vi "crosscorr_sub2.vi"(0 "reference":refnum<vi>, 1 "B":dbl=500.0 format="%.2f", 5 "binning":refnum<vi>, 7 "macro times 1":i32[](array[numeric]), 9 "macro times 2":i32[](array[numeric]), 11 "cross ch2 (MCS)":i32, 12 "cross ch1 (MCS)":i32, 13 "skip":i32, 14 "biExp fit":bool) -> (6 "crosscorrelation":cluster{"Tau Values":dbl[], "best fit":dbl[]}[](array[cluster]), 8 "F2":dbl, 10 "S+B":dbl, 15 "fit results":cluster{dbl, dbl, dbl, dbl, dbl, dbl})   [LabVIEW 2009]
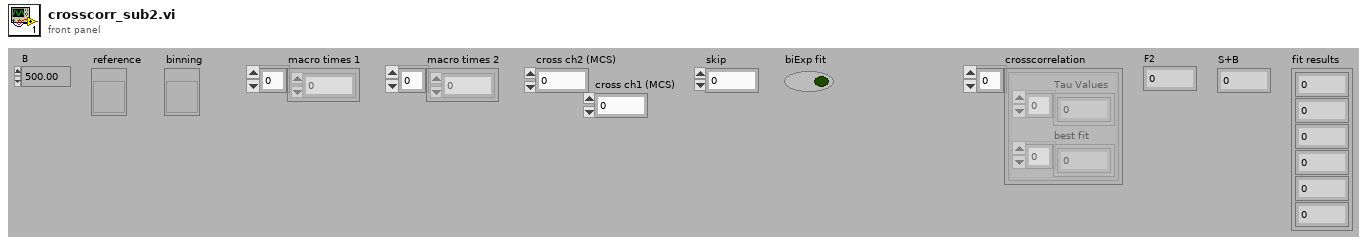
[diagram p1: front panel]
types:
  T1 = cluster{"binning (s)":dbl, "binning (s)":dbl, "Histogram: h(x)":u32[]}[]
  T2 = cluster{"binning (s)":dbl, "binning (s)":dbl, "Histogram: h(x)":u32[]}
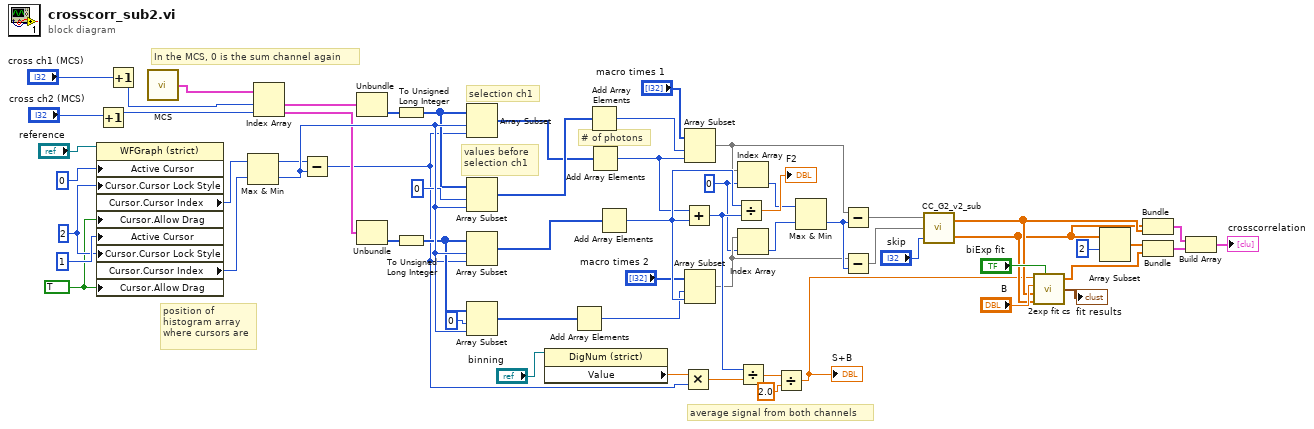
[diagram p0: block diagram]
diagram:
  w39 = 0 ("Index")
  w23 = u32 2 ("Write Attribute")
  w16 = TRUE ("Write Attribute")
  # "average signal from both channels"
  # "In the MCS, 0 is the sum channel again"
  # "# of photons"
  # "values before \nselection ch1"
  # "position of\nhistogram array\nwhere cursors are"
  # "selection ch1"
  n1 = property on="Property Node" class="WFGraph (strict)"(reference="reference", "Active Cursor"=u32 0, "Cursor.Cursor Lock Style"=w23, "Cursor.Allow Drag"=w16, "Active Cursor"=u32 1, "Cursor.Cursor Lock Style"=w23, "Cursor.Allow Drag"=w16) -> ("Cursor.Cursor Index"=w17:i32, "Cursor.Cursor Index"=w18:i32)  [unwired: 1 in, 2 out]
  n2 = Increment(x="cross ch2 (MCS)") -> (x+1=w4:i32)
  n3 = Increment(x="cross ch1 (MCS)") -> (x+1=w6:i32)
  n4 = call "MCS.vi"() -> ("MCS output"=w26:T1)  [unwired: 2 in]
  n5 = Max & Min(x=w17, y=w18) -> (max(x,y)=w27:i32, min(x,y)=w32:i32)
  n6 = Index Array(array=w26, index #1=w6, index #2=w4) -> (element #1=w8:T2, element #2=w28:T2)
  n7 = Subtract(x=w27, y=w32) -> (x-y=w10:i32)
  n8 = Unbundle(w8) -> ("Histogram: h(x)"=w22:u32[])  [unwired: 2 out]
  n9 = Unbundle(w28) -> ("Histogram: h(x)"=w29:u32[])  [unwired: 2 out]
  n10 = To Unsigned Long Integer(number=w22) -> (unsigned 32bit integer=w20:u32[])
  n11 = To Unsigned Long Integer(number=w29) -> (unsigned 32bit integer=w30:u32[])
  n12 = Array Subset(array=w20, index=w32, length=w10) -> (w15:u32[])
  n13 = Array Subset(array=w20, index=0, length=w32) -> (w19:u32[])
  n14 = Array Subset(array=w30, index=w32, length=w10) -> (w34:u32[])
  n15 = Array Subset(array=w30, index=0, length=w32) -> (w33:u32[])
  n16 = property class="DigNum (strict)"(reference="binning") -> ("Value"=w47:dbl)  [unwired: 1 in, 2 out]
  n17 = Add Array Elements(numeric array=w33) -> (sum=w35:u32)
  n18 = Add Array Elements(numeric array=w19) -> (sum=w21:u32)
  n19 = Add Array Elements(numeric array=w15) -> (sum=w48:u32)
  n20 = Add Array Elements(numeric array=w34) -> (sum=w50:u32)
  n21 = Multiply(x=w47, y=w10) -> (x*y=w49:dbl)
  n22 = Add(x=w48, y=w50) -> (x+y=w51:u32)
  n23 = Array Subset(array="macro times 1", index=w21, length=w48) -> (w36:i32[])
  n24 = Array Subset(array="macro times 2", index=w35, length=w50) -> (w40:i32[])
  n25 = Divide(x=w50, y=w51) -> (x/y=→"F2":dbl)
  n26 = Index Array(array=w36, index=w39) -> (element=w41:i32)
  n27 = Index Array(array=w40, index=w39) -> (element=w42:i32)
  n28 = Divide(x=w51, y=w49) -> (x/y=w3:dbl)
  n29 = Divide(x=w3, y=2.0) -> (x/y=w2:dbl)
  "S+B" <- w2
  n30 = Max & Min(x=w41, y=w42) -> (min(x,y)=w43:i32)  [unwired: 1 out]
  n31 = Subtract(x=w36, y=w43) -> (x-y=w59:i32[])
  n32 = Subtract(x=w40, y=w43) -> (x-y=w60:i32[])
  n33 = call "CC_G2_v2_sub.vi"("skip n"="skip", "Macros2"=w60, "Macros1"=w59) -> ("Tau Values"=w54:dbl[], "G2 vals"=w55:dbl[])
  n34 = call "2exp fit cs.vi"("S+B"=w2, "biExp fit"="biExp fit", "B"="B", "y"=w55, "x"=w54) -> ("best fit"=w53:dbl[], "results"=→"fit results":cluster{dbl, dbl, dbl, dbl, dbl, dbl})  [unwired: 1 in, 1 out]
  n35 = Array Subset(array=w54, index=2) -> (w46:dbl[])  [unwired: 1 in]
  n36 = Bundle("Tau Values"=w54, "G2 vals"=w55) -> (w37:cluster{"Tau Values":dbl[], "G2 vals":dbl[]})  [unwired: 1 in]
  n37 = Bundle(w46, "best fit"=w53) -> (w44:cluster{dbl[], "best fit":dbl[]})  [unwired: 1 in]
  n38 = Build Array(w37, w44) -> (→"crosscorrelation":cluster{"Tau Values":dbl[], "best fit":dbl[]}[])
